vi "Set Position Setpoint.vi"(8 "error in (no error)":errorcluster, 10 "CCW position (rad)":dbl, 11 "simulated KUKA youBot arm motor in":refnum<class "NI_Robotics_KUKA youBot Arm Motor_Sim.lvclass">) -> (0 "error out":errorcluster, 3 "simulated KUKA youBot arm motor out":refnum<class "NI_Robotics_KUKA youBot Arm Motor_Sim.lvclass">)   [LabVIEW 2017, in "NI_Robotics_KUKA youBot Host.lvlib" / "NI_Robotics_KUKA youBot Arm Motor_Sim.lvclass"]
uses:
  <vilib>/robotics/KUKA youBot/Motor/Arm Motor Sim/NI_Robotics_KUKA youBot Arm Motor_Sim.lvclass
  c:/Program Files (x86)/National Instruments/LabVIEW 2017/vi.lib/robotics/KUKA youBot/Motor/Arm Motor/NI_Robotics_KUKA youBot Arm Motor.lvclass
  <vilib>/robotics/KUKA youBot/Motor/Arm Motor Sim/NI_Robotics_KUKA youBot Arm Motor_Sim.lvclass/NI_Robotics_KUKA youBot Arm Motor_Sim.ctl
  <vilib>/robotics/Simulator/Robot Factory/Motor/ODESimulator_Motor.lvclass
  <vilib>/robotics/KUKA youBot/Motor/Arm Motor/NI_Robotics_KUKA youBot Arm Motor.lvclass
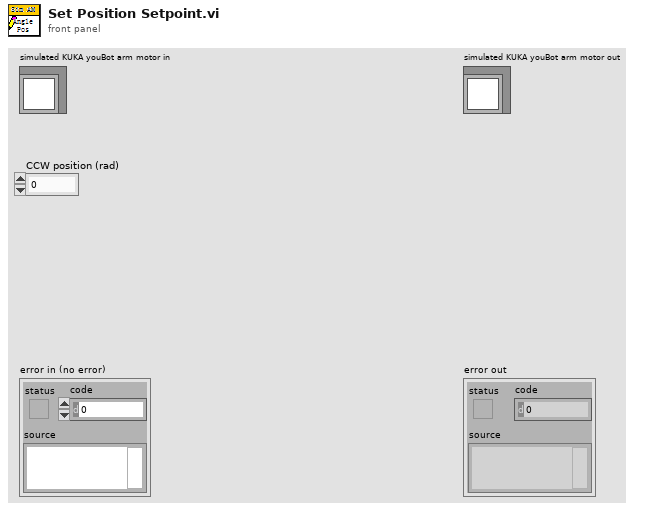
[diagram p1: front panel]
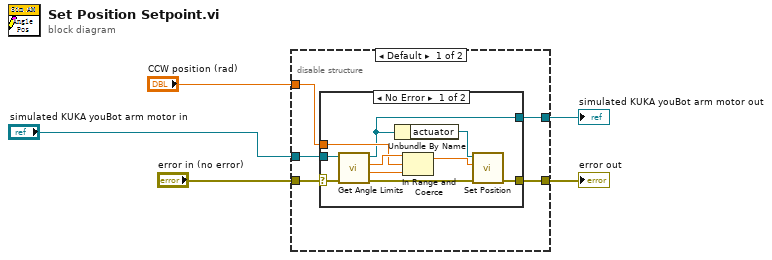
[diagram p0: block diagram]
diagram:
  n1 = disable-structure shown="Default" {
    disable-tunnel: "error in (no error)" -> [w10 w23]
    disable-tunnel: "CCW position (rad)" -> [w9 _]
    disable-tunnel: "simulated KUKA youBot arm motor in" -> [w8 w24]
    disable-tunnel: [w7 w23] -> w2
    disable-tunnel: [w6 w24] -> w1
    frame condition #0 (active) {
      n2 = case shown="No Error" w10 {
        selector: w10 -> [w19 w21]
        tunnel: w9 -> [w16 _]
        tunnel: w8 -> [w20 w22]
        tunnel: [w13 w21] -> w7
        tunnel: [w15 w22] -> w6
        frame No Error {
          n3 = call <vilib>:"Get Angle Limits.vi"("error in (no error)"=w19, "KUKA youBot arm motor in"=w20) -> ("error out"=w14:errorcluster, "min angle (rad)"=w17:dbl, "max angle (rad)"=w18:dbl, "KUKA youBot arm motor out"=w15:refnum<class "NI_Robotics_KUKA youBot Arm Motor_Sim.lvclass">)  [unwired: 6 in]
          n4 = Unbundle By Name(w15) -> ("actuator"=w11:refnum<class "ODESimulator_Motor.lvclass">)
          n5 = In Range and Coerce(upper limit=w18, x=w16, lower limit=w17) -> (coerced(x)=w12:dbl)  [unwired: 1 out]
          n6 = call-dynamic "Set Position.vi"("error in (no error)"=w14, "CCW Position (0.0 rad)"=w12, "Motor in"=w11) -> ("error out"=w13:errorcluster)  [unwired: 7 in, 1 out]
        }
        frame Error {
        }
      }
    }
    frame condition #1 {
    }
  }
  "error out" <- w2
  "simulated KUKA youBot arm motor out" <- w1
